vi "Begin.vi"(8 "error in":errorcluster) -> (0 "error out":errorcluster)   [LabVIEW 2018]
doc: "Called before other user functions, this VI is expected to open initial I/O refnums, load in file data, and do all program initialization. Notice that the <B>error out</B> terminal is simply used for data flow. Wiring it to other structures or subVIs ensures that this VI runs first."
uses:
  <vilib>/Rock Robotics/WPI/DriverStation/WPI_DriverStationRobotMode2.ctl
  <vilib>/Rock Robotics/WPI/Joystick/WPI_JoystickDeviceEnum.ctl
  <vilib>/Rock Robotics/SystemInterfaces/AI/FPGA_AIChannel.ctl
  <vilib>/Rock Robotics/SystemInterfaces/spilib/spi_bus.ctl
  Robot Global Data.vi
  Swerve/SwerveGlobals.vi
  navx-mxp/labview/navX Library v2/IO/Open/Z900_navX_Open_SPI.vi
  navx-mxp/labview/navX Library v2/navX Library v2.lvlib
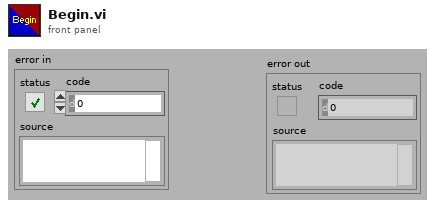
[diagram p1: front panel]
types:
  T1 = typedef "WPI_DriverStationRobotMode2.ctl" = enum16{"Autonomous Disabled", "Autonomous Enabled", "Teleop Disabled", "Teleop Enabled", "Disconnected", "Finish", "Test Disabled", "Test Enabled", "Emergency Stopped"}
  T2 = typedef "WPI_JoystickDeviceEnum.ctl" = enum16{"USB 0", "USB 1", "USB 2", "USB 3", "USB 4", "USB 5"}
  T3 = typedef "FPGA_AIChannel.ctl" = enum8{"AI 0", "AI 1", "AI 2", "AI 3", "AI MXP 0", "AI MXP 1", "AI MXP 2", "AI MXP 3", "Invalid"}
  T4 = typedef "spi_bus.ctl" = enum16{"SPI On-Board, CS0", "SPI On-Board, CS1", "SPI On-Board, CS2", "SPI On-Board, CS3", "SPI MXP", "Invalid"}
  T5 = typedef "WPI_JoystickDevRef.ctl" = cluster{"Device":T2}
  T6 = typedef "WPI_MotorControlDeviceRef.ctl" = cluster{"DeviceStatus":errorcluster, "Type":T7, "PWM":cluster{"PWM Channel":T8, "DeadBand":T9}, "CAN":cluster{"Device Number":u8, "SetOutput VI Ref":variant, "GetOutput VI Ref":variant, "Enable VI Ref":variant, "Disable VI Ref":variant, "Data":variant}, "Invert":bool, "DIO PWM":cluster{"PWM \"Enable\" Channel":T8, "DIOChannel":T10, "PWM Rate":dbl}}
  T7 = typedef "WPI_MotorControlType.ctl" = enum16{"PWM", "CAN", "DIO PWM"}
  T8 = typedef "FPGA_DIOPWMChannel.ctl" = enum8{"PWM 0", "PWM 1", "PWM 2", "PWM 3", "PWM 4", "PWM 5", "PWM 6", "PWM 7", "PWM 8", "PWM 9", "PWM MXP 0", "PWM MXP 1", "PWM MXP 2", "PWM MXP 3", "PWM MXP 4", "PWM MXP 5", "PWM MXP 6", "PWM MXP 7", "PWM MXP 8", "PWM MXP 9", "Invalid"}
  T9 = typedef "WPI_PWMDeadband.ctl" = cluster{"Name":string, "maxPositivePwm":i32, "minPositivePwm":i32, "centerPwm":i32, "maxNegativePwm":i32, "minNegativePwm":i32, "angularRange":u16}
  T10 = typedef "FPGA_DIOChannel.ctl" = enum8{"DIO 0", "DIO 1", "DIO 2", "DIO 3", "DIO 4", "DIO 5", "DIO 6", "DIO 7", "DIO 8", "DIO 9", "DIO MXP 0", "DIO MXP 1", "DIO MXP 2", "DIO MXP 3", "DIO MXP 4", "DIO MXP 5", "DIO MXP 6", "DIO MXP 7", "DIO MXP 8", "DIO MXP 9", "DIO MXP 10", "DIO MXP 11", "DIO MXP 12", "DIO MXP 13", "DIO MXP 14", "DIO MXP 15", "SPI Port CS1", "SPI Port CS2", "SPI Port CS3", "SPI Port MISO", "SPI Port MOSI", "Invalid"}
  T11 = typedef "WPI_AnalogChannelDevRef.ctl" = cluster{"DevStatus":errorcluster, "Analog Channel":T3}
  T12 = typedef "navX Library v2.lvlib/Z900_navX_DeviceTypeDef.ctl" = cluster{"Interface":cluster{"Protocol":T13, "Update Rate (4Hz-100Hz)":u8, "navX Open TypeDef":variant}, "Notify Packet":refnum<notifier>, "Loop VI Refnum":refnum<vi>, "Ready to Close Occurrence Refnum":refnum<k4>}
  T13 = typedef "navX Library v2.lvlib/Z900_navX_ProtocolTypeDef.ctl" = enum16{"SERIAL", "I2C", "SPI"}
  T14 = cluster{"Yaw":dbl, "Roll":dbl, "Pitch":dbl, "Heading":dbl, "Fused Heading":dbl}
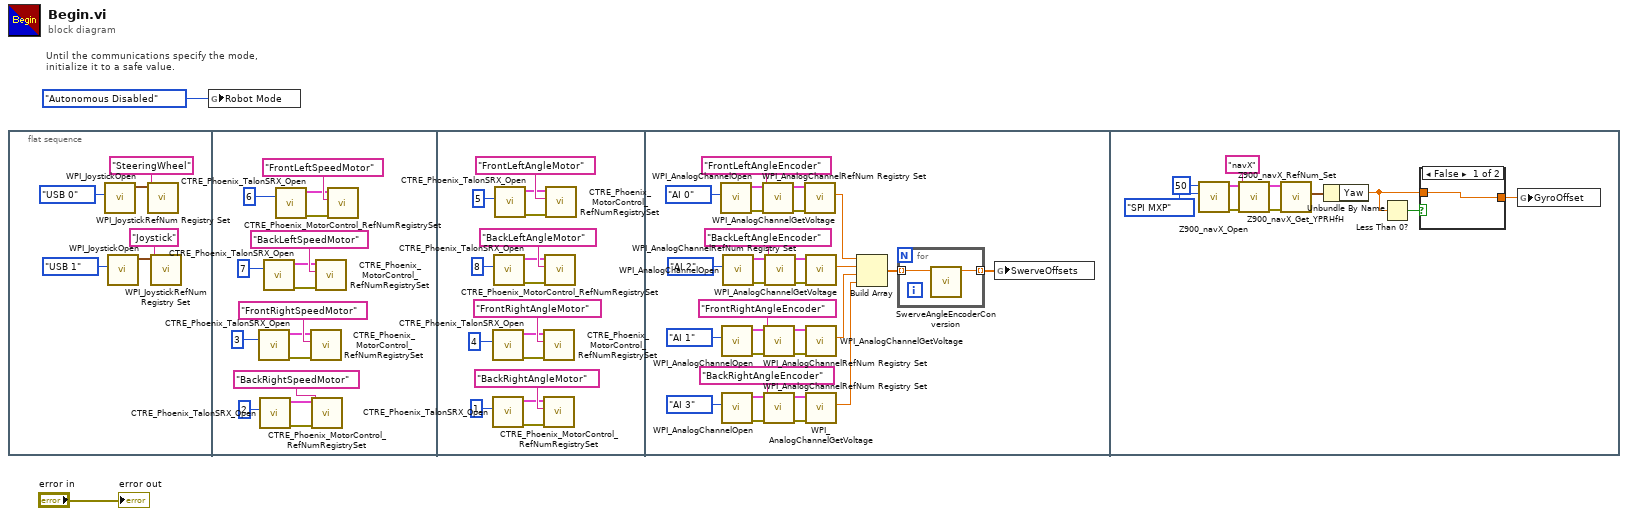
[diagram p0: block diagram]
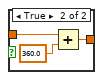
[diagram p2: hidden frame]
diagram:
  # "Until the communications specify the mode,\ninitialize it to a safe value."
  n1 = flat-sequence {
    frame #0 {
      n2 = call <vilib>:"WPI_JoystickOpen.vi"("JoystickDevice"=WPI_JoystickDeviceEnum."USB 0") -> ("JoystickDevRef"=w8:T5)  [unwired: 10 in]
      n3 = call <vilib>:"WPI_JoystickOpen.vi"("JoystickDevice"=WPI_JoystickDeviceEnum."USB 1") -> ("JoystickDevRef"=w5:T5)  [unwired: 10 in]
      n4 = call <vilib>:"WPI_JoystickRefNum Registry Set.vi"("refnum name"="SteeringWheel", "JoystickDevRef"=w8) -> ()  [unwired: 8 in, 2 out]
      n5 = call <vilib>:"WPI_JoystickRefNum Registry Set.vi"("refnum name"="Joystick", "JoystickDevRef"=w5) -> ()  [unwired: 8 in, 2 out]
    }
    frame #1 {
      n6 = call <vilib>:"CTRE_Phoenix_TalonSRX_Open.vi"("Device Number"=u8 3) -> ("error out"=w13:errorcluster, "CAN Talon SRX Ref"=w14:T6)  [unwired: 9 in]
      n7 = call <vilib>:"CTRE_Phoenix_TalonSRX_Open.vi"("Device Number"=u8 2) -> ("error out"=w15:errorcluster, "CAN Talon SRX Ref"=w16:T6)  [unwired: 9 in]
      n8 = call <vilib>:"CTRE_Phoenix_TalonSRX_Open.vi"("Device Number"=u8 7) -> ("error out"=w11:errorcluster, "CAN Talon SRX Ref"=w12:T6)  [unwired: 9 in]
      n9 = call <vilib>:"CTRE_Phoenix_TalonSRX_Open.vi"("Device Number"=u8 6) -> ("error out"=w9:errorcluster, "CAN Talon SRX Ref"=w10:T6)  [unwired: 9 in]
      n10 = call <vilib>:"CTRE_Phoenix_MotorControl_RefNumRegistrySet.vi"("error in (no error)"=w13, "refnum name"="FrontRightSpeedMotor", "PhoenixMotorControlDevRef"=w14) -> ()  [unwired: 7 in, 2 out]
      n11 = call <vilib>:"CTRE_Phoenix_MotorControl_RefNumRegistrySet.vi"("error in (no error)"=w15, "refnum name"="BackRightSpeedMotor", "PhoenixMotorControlDevRef"=w16) -> ()  [unwired: 7 in, 2 out]
      n12 = call <vilib>:"CTRE_Phoenix_MotorControl_RefNumRegistrySet.vi"("error in (no error)"=w11, "refnum name"="BackLeftSpeedMotor", "PhoenixMotorControlDevRef"=w12) -> ()  [unwired: 7 in, 2 out]
      n13 = call <vilib>:"CTRE_Phoenix_MotorControl_RefNumRegistrySet.vi"("error in (no error)"=w9, "refnum name"="FrontLeftSpeedMotor", "PhoenixMotorControlDevRef"=w10) -> ()  [unwired: 7 in, 2 out]
    }
    frame #2 {
      n14 = call <vilib>:"CTRE_Phoenix_TalonSRX_Open.vi"("Device Number"=u8 4) -> ("error out"=w27:errorcluster, "CAN Talon SRX Ref"=w28:T6)  [unwired: 9 in]
      n15 = call <vilib>:"CTRE_Phoenix_TalonSRX_Open.vi"("Device Number"=u8 1) -> ("error out"=w25:errorcluster, "CAN Talon SRX Ref"=w26:T6)  [unwired: 9 in]
      n16 = call <vilib>:"CTRE_Phoenix_TalonSRX_Open.vi"("Device Number"=u8 8) -> ("error out"=w29:errorcluster, "CAN Talon SRX Ref"=w30:T6)  [unwired: 9 in]
      n17 = call <vilib>:"CTRE_Phoenix_TalonSRX_Open.vi"("Device Number"=u8 5) -> ("error out"=w31:errorcluster, "CAN Talon SRX Ref"=w32:T6)  [unwired: 9 in]
      n18 = call <vilib>:"CTRE_Phoenix_MotorControl_RefNumRegistrySet.vi"("error in (no error)"=w27, "refnum name"="FrontRightAngleMotor", "PhoenixMotorControlDevRef"=w28) -> ()  [unwired: 7 in, 2 out]
      n19 = call <vilib>:"CTRE_Phoenix_MotorControl_RefNumRegistrySet.vi"("error in (no error)"=w25, "refnum name"="BackRightAngleMotor", "PhoenixMotorControlDevRef"=w26) -> ()  [unwired: 7 in, 2 out]
      n20 = call <vilib>:"CTRE_Phoenix_MotorControl_RefNumRegistrySet.vi"("error in (no error)"=w29, "refnum name"="BackLeftAngleMotor", "PhoenixMotorControlDevRef"=w30) -> ()  [unwired: 7 in, 2 out]
      n21 = call <vilib>:"CTRE_Phoenix_MotorControl_RefNumRegistrySet.vi"("error in (no error)"=w31, "refnum name"="FrontLeftAngleMotor", "PhoenixMotorControlDevRef"=w32) -> ()  [unwired: 7 in, 2 out]
    }
    frame #3 {
      n22 = call <vilib>:"WPI_AnalogChannelOpen.vi"("Analog Channel"=FPGA_AIChannel."AI 0") -> ("error out"=w69:errorcluster, "AIDeviceRef"=w70:T11)  [unwired: 9 in]
      n23 = call <vilib>:"WPI_AnalogChannelOpen.vi"("Analog Channel"=FPGA_AIChannel."AI 1") -> ("error out"=w61:errorcluster, "AIDeviceRef"=w62:T11)  [unwired: 9 in]
      n24 = call <vilib>:"WPI_AnalogChannelOpen.vi"("Analog Channel"=FPGA_AIChannel."AI 3") -> ("error out"=w57:errorcluster, "AIDeviceRef"=w58:T11)  [unwired: 9 in]
      n25 = call <vilib>:"WPI_AnalogChannelOpen.vi"("Analog Channel"=FPGA_AIChannel."AI 2") -> ("error out"=w65:errorcluster, "AIDeviceRef"=w66:T11)  [unwired: 9 in]
      n26 = call <vilib>:"WPI_AnalogChannelRefNum Registry Set.vi"("error in (no error)"=w69, "refnum name"="FrontLeftAngleEncoder", "AIDeviceRef"=w70) -> ("error out"=w53:errorcluster, "AIDeviceRef"=w54:T11)  [unwired: 7 in]
      n27 = call <vilib>:"WPI_AnalogChannelRefNum Registry Set.vi"("error in (no error)"=w61, "refnum name"="FrontRightAngleEncoder", "AIDeviceRef"=w62) -> ("error out"=w49:errorcluster, "AIDeviceRef"=w50:T11)  [unwired: 7 in]
      n28 = call <vilib>:"WPI_AnalogChannelRefNum Registry Set.vi"("error in (no error)"=w57, "refnum name"="BackRightAngleEncoder", "AIDeviceRef"=w58) -> ("error out"=w47:errorcluster, "AIDeviceRef"=w48:T11)  [unwired: 7 in]
      n29 = call <vilib>:"WPI_AnalogChannelRefNum Registry Set.vi"("error in (no error)"=w65, "refnum name"="BackLeftAngleEncoder", "AIDeviceRef"=w66) -> ("error out"=w51:errorcluster, "AIDeviceRef"=w52:T11)  [unwired: 7 in]
      n30 = call <vilib>:"WPI_AnalogChannelGetVoltage.vi"("error in (no error)"=w53, "AIDeviceRef"=w54) -> ("Voltage"=w46:dbl)  [unwired: 7 in, 2 out]
      n31 = call <vilib>:"WPI_AnalogChannelGetVoltage.vi"("error in (no error)"=w51, "AIDeviceRef"=w52) -> ("Voltage"=w45:dbl)  [unwired: 7 in, 2 out]
      n32 = call <vilib>:"WPI_AnalogChannelGetVoltage.vi"("error in (no error)"=w49, "AIDeviceRef"=w50) -> ("Voltage"=w44:dbl)  [unwired: 7 in, 2 out]
      n33 = call <vilib>:"WPI_AnalogChannelGetVoltage.vi"("error in (no error)"=w47, "AIDeviceRef"=w48) -> ("Voltage"=w43:dbl)  [unwired: 7 in, 2 out]
      n34 = Build Array(w46, w45, w44, w43) -> (w42:dbl[])
      n35 = for {
        tunnel: w42 -> [w72] mode=indexing
        tunnel: [w71] -> w41 mode=indexing
        n36 = call "SwerveAngleEncoderConversion.vi"("Voltage"=w72) -> ("Angle"=w71:dbl)  [unwired: 10 in]
      }
      n37 = global write "SwerveGlobals.vi" "SwerveOffsets"(w41) -> ()
    }
    frame #4 {
      n38 = call-poly "Z900_navX_Open.vi"("SPI Bus"=spi_bus."SPI MXP", "Update Rate (4Hz-60Hz)"=u8 50) -> ("error out"=w83:errorcluster, "navX Device"=w82:T12)  [unwired: 8 in]
      n39 = call "Z900_navX_RefNum_Set.vi"("error in (no error)"=w83, "refnum name"="navX", "navX Device"=w82) -> ("error out"=w76:errorcluster, "navX Device"=w77:T12)  [unwired: 7 in]
      n40 = call "Z900_navX_Get_YPRHfH.vi"("error in (no error)"=w76, "navX Device"=w77) -> ("YRPHfH"=w78:T14)  [unwired: 6 in, 3 out]
      n41 = Unbundle By Name(w78) -> ("Yaw"=w74:dbl)
      n42 = Less Than 0?(x=w74) -> (x < 0?=w75:bool)
      n43 = case shown="False" w75 {
        tunnel: w74 -> [w84 w87]
        tunnel: [w84 w85] -> w73
        frame False {
        }
        frame True {
          n44 = Add(x=w87, y=360.0) -> (x+y=w85:dbl)
        }
      }
      n45 = global write "SwerveGlobals.vi" "GyroOffset"(w73) -> ()
    }
  }
  n46 = global write "Robot Global Data.vi" "Robot Mode"(WPI_DriverStationRobotMode2."Autonomous Disabled" ("Robot Mode")) -> ()
  "error out" <- "error in"
